vi "Table_Operation.vi"() -> ()   [LabVIEW 2009]
panel:
  in  "stop":bool
  in  "1D Array":string[](array[string])
  in  "Multicolumn Listbox":i32(listbox)
  in  "Remove":bool
  in  "Add":bool
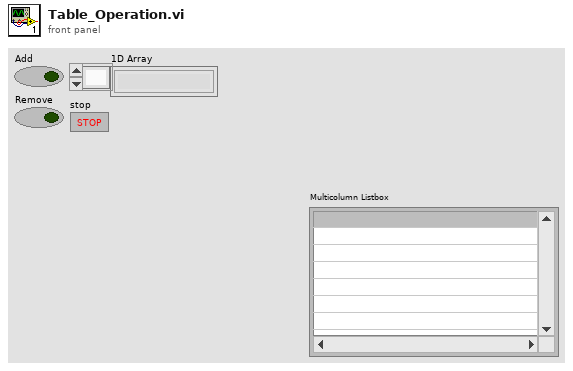
[diagram p1: front panel]
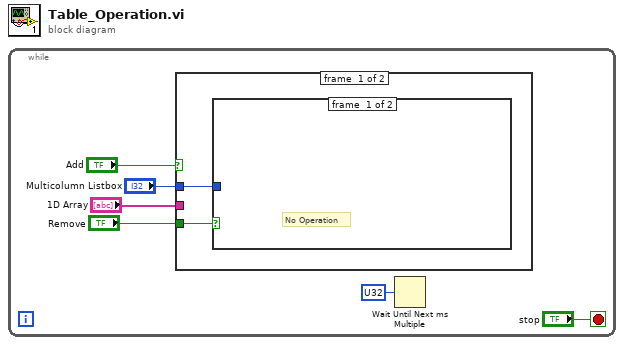
[diagram p0: block diagram]
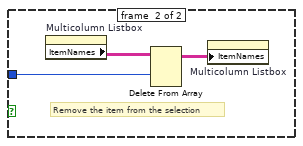
[diagram p2: hidden frame]
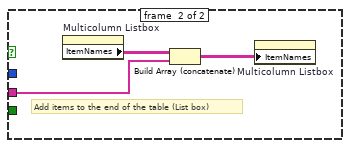
[diagram p3: hidden frame]
diagram:
  n1 = while {
    stop <- "stop" stop-if-true
    n2 = case shown="True" "Add" {
      tunnel: "1D Array" -> [_ w13]
      tunnel: "Multicolumn Listbox" -> [w7 _]
      tunnel: "Remove" -> [w8 _]
      frame #0 {
        n3 = case shown="True" w8 {
          tunnel: w7 -> [_ w10]
          frame #0 {
            # "No Operation"
          }
          frame #1 {
            # "Remove the item from the selection"
            n4 = property on="Multicolumn Listbox" class="MCListbox (strict)"() -> ("ItemNames"=w11:string[][])  [unwired: 2 in, 2 out]
            n5 = Delete From Array(array=w11, index (row)=w10) -> (array with subset deleted=w9:string[][])  [unwired: 2 in, 1 out]
            n6 = property on="Multicolumn Listbox" class="MCListbox (strict)"("ItemNames"=w9) -> ()  [unwired: 2 in, 2 out]
          }
        }
      }
      frame #1 {
        # "Add items to the end of the table (List box)"
        n7 = property on="Multicolumn Listbox" class="MCListbox (strict)"() -> ("ItemNames"=w14:string[][])  [unwired: 2 in, 2 out]
        n8 = Build Array (concatenate)(w14, w13) -> (w12:string[][])
        n9 = property on="Multicolumn Listbox" class="MCListbox (strict)"("ItemNames"=w12) -> ()  [unwired: 2 in, 2 out]
      }
    }
    n10 = Wait Until Next ms Multiple(millisecond multiple=u32 ?) -> ()  [unwired: 1 out]
  }
